vi "Recipe XML Editor.vi"(11 "TopLevel In":refnum<class "TopLevel.lvclass">) -> (3 "TopLevel out":refnum<class "TopLevel.lvclass">)   [LabVIEW 2022 SP3, in "TopLevel.lvclass"]
uses:
  TopLevel.lvclass
  Common/Controls/DLP2RecipeV2.ctl
panel:
  in  "Save Data to Recipe XML":bool
  in  "DLP":T1
  in  "Read Recipe XML":bool
  in  "Recipe XML File Path":path
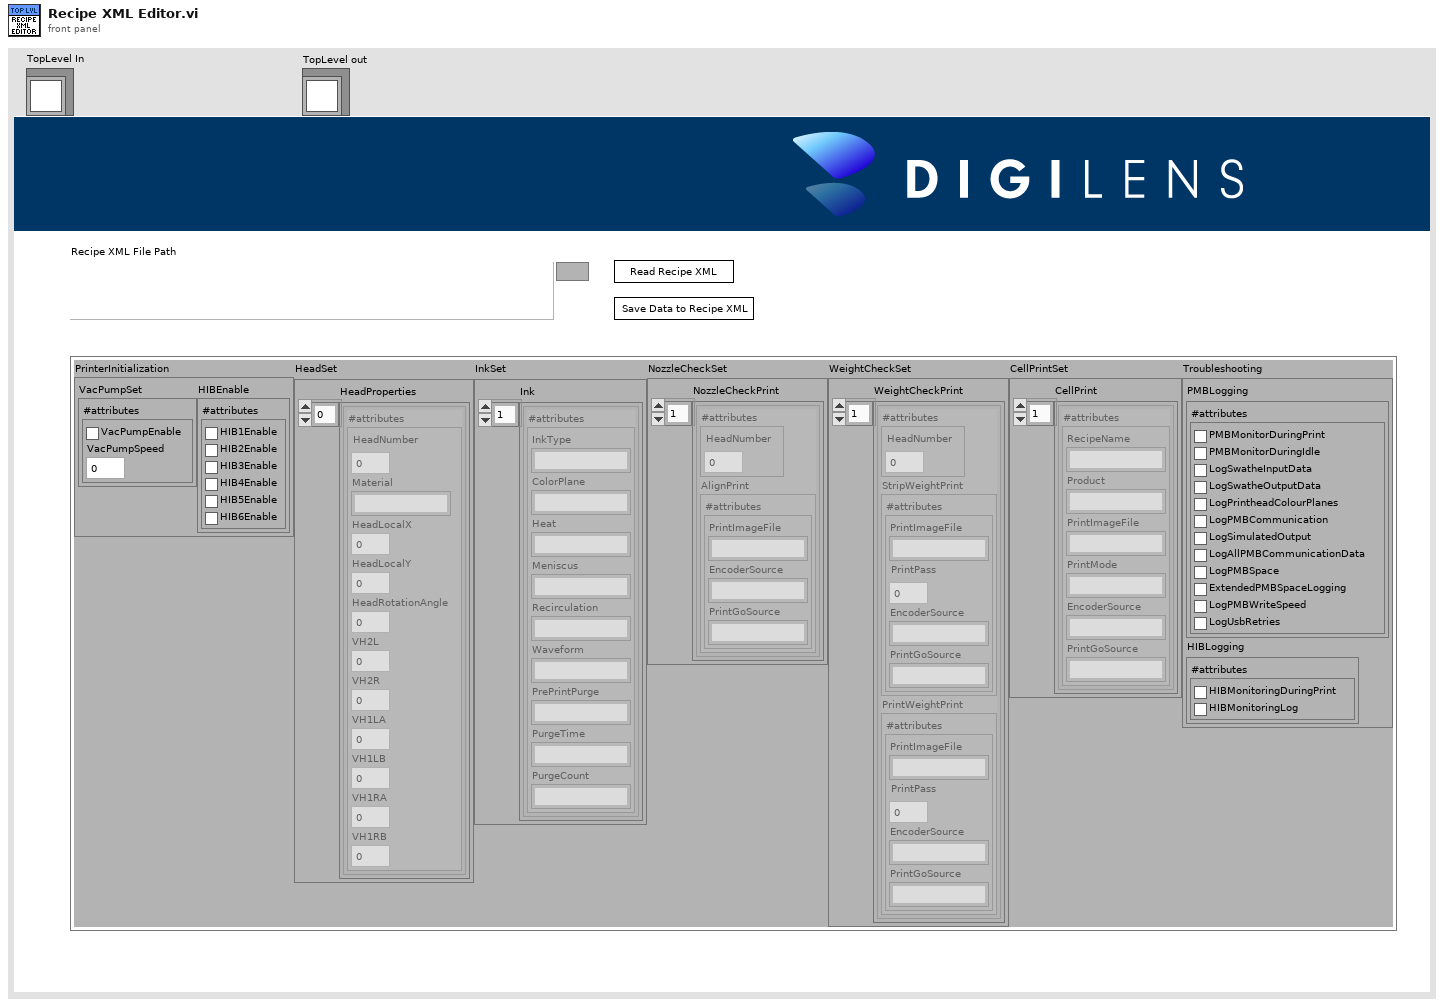
[diagram p1: front panel]
types:
  T1 = typedef "DLP2RecipeV2.ctl" = cluster{"PrinterInitialization":cluster{"VacPumpSet":cluster{"#attributes":cluster{"VacPumpEnable":bool, "VacPumpSpeed":dbl}}, "HIBEnable":cluster{"#attributes":cluster{"HIB1Enable":bool, "HIB2Enable":bool, "HIB3Enable":bool, "HIB4Enable":bool, "HIB5Enable":bool, "HIB6Enable":bool}}}, "HeadSet":cluster{"HeadProperties":cluster{"#attributes":cluster{"HeadNumber":u8, "Material":string, "HeadLocalX":dbl, "HeadLocalY":dbl, "HeadRotationAngle":dbl, "VH2L":dbl, "VH2R":dbl, "VH1LA":dbl, "VH1LB":dbl, "VH1RA":dbl, "VH1RB":dbl}}[]}, "InkSet":cluster{"Ink":cluster{"#attributes":cluster{"InkType":string, "ColorPlane":string, "Heat":string, "Meniscus":string, "Recirculation":string, "Waveform":string, "PrePrintPurge":string, "PurgeTime":string, "PurgeCount":string}}[]}, "NozzleCheckSet":cluster{"NozzleCheckPrint":cluster{"#attributes":cluster{"HeadNumber":u8}, "AlignPrint":cluster{"#attributes":cluster{"PrintImageFile":string, "EncoderSource":string, "PrintGoSource":string}}}[]}, "WeightCheckSet":cluster{"WeightCheckPrint":cluster{"#attributes":cluster{"HeadNumber":u8}, "StripWeightPrint":cluster{"#attributes":cluster{"PrintImageFile":string, "PrintPass":u8, "EncoderSource":string, "PrintGoSource":string}}, "PrintWeightPrint":cluster{"#attributes":cluster{"PrintImageFile":string, "PrintPass":u8, "EncoderSource":string, "PrintGoSource":string}}}[]}, "CellPrintSet":cluster{"CellPrint":cluster{"#attributes":cluster{"RecipeName":string, "Product":string, "PrintImageFile":string, "PrintMode":string, "EncoderSource":string, "PrintGoSource":string}}[]}, "Troubleshooting":cluster{"PMBLogging":cluster{"#attributes":cluster{"PMBMonitorDuringPrint":bool, "PMBMonitorDuringIdle":bool, "LogSwatheInputData":bool, "LogSwatheOutputData":bool, "LogPrintheadColourPlanes":bool, "LogPMBCommunication":bool, "LogSimulatedOutput":bool, "LogAllPMBCommunicationData":bool, "LogPMBSpace":bool, "ExtendedPMBSpaceLogging":bool, "LogPMBWriteSpeed":bool, "LogUsbRetries":bool}}, "HIBLogging":cluster{"#attributes":cluster{"HIBMonitoringDuringPrint":bool, "HIBMonitoringLog":bool}}}}
  T2 = enum32{"invalid app kind", "Development System", "Run Time System", "Student Edition", "Embedded LabVIEW", "Evaluation", "Custom"}
  T3 = enum32{"Invalid", "Standard", "Closed", "Hidden", "Minimized", "Maximized"}
  T4 = cluster{"Core":cluster{"Current VI Reference":refnum<vi>, "Close Panel on Exit?":bool}, "TopLevel In":refnum<class "TopLevel.lvclass">}
  T5 = cluster{"Current VI Reference":refnum<vi>, "Close Panel on Exit?":bool}
  T6 = typedef "TopLevel.lvclass/UserEvents.ctl" = cluster{"API Incoming Event":refnum<user-event>, "API Executed Event":refnum<user-event>, "API Return Event":refnum<user-event>, "Exit Event":refnum<user-event>, "StatusChanged":refnum<user-event>, "DLP GUI Config Changed":refnum<user-event>, "AppEvent":refnum<user-event>, "Login Event":refnum<user-event>, "HeadPrimeStatusEvent":refnum<user-event>}
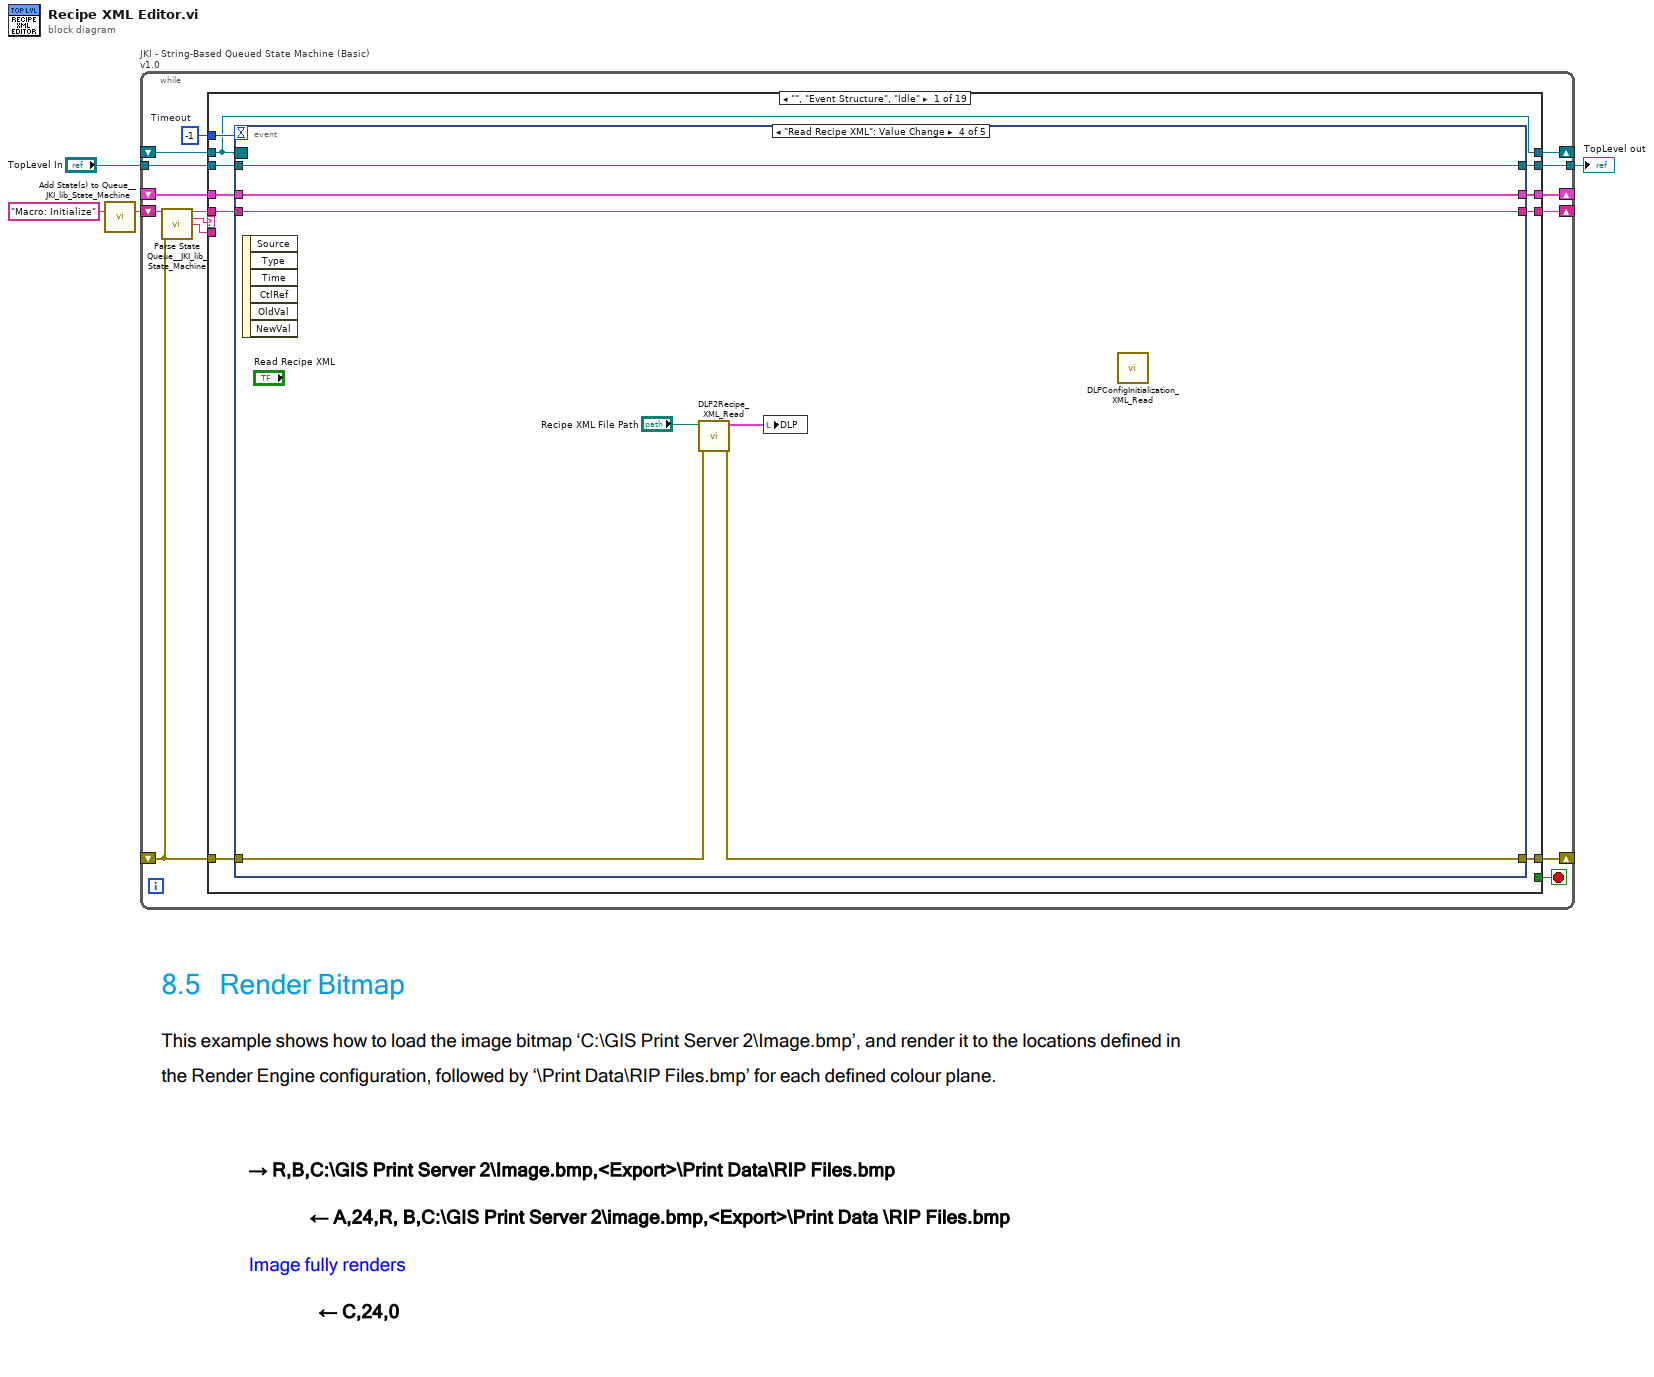
[diagram p0: block diagram]
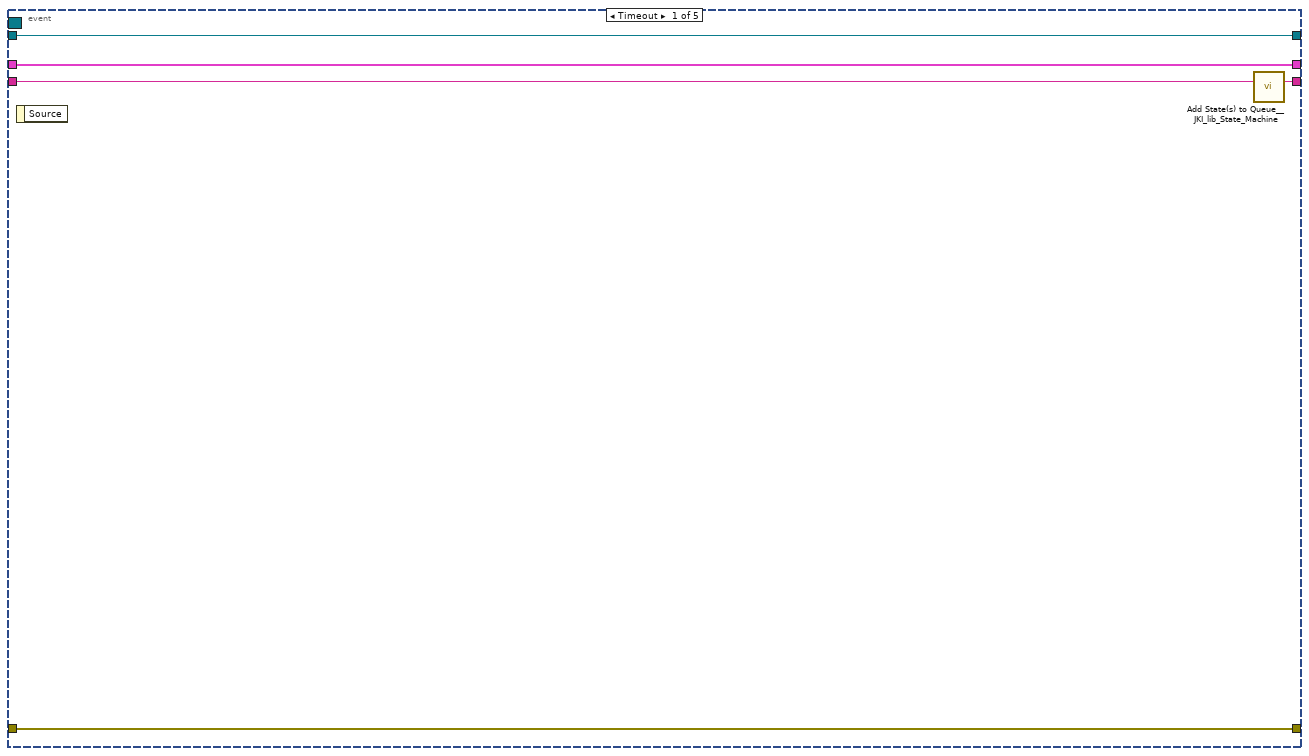
[diagram p2: hidden frame]
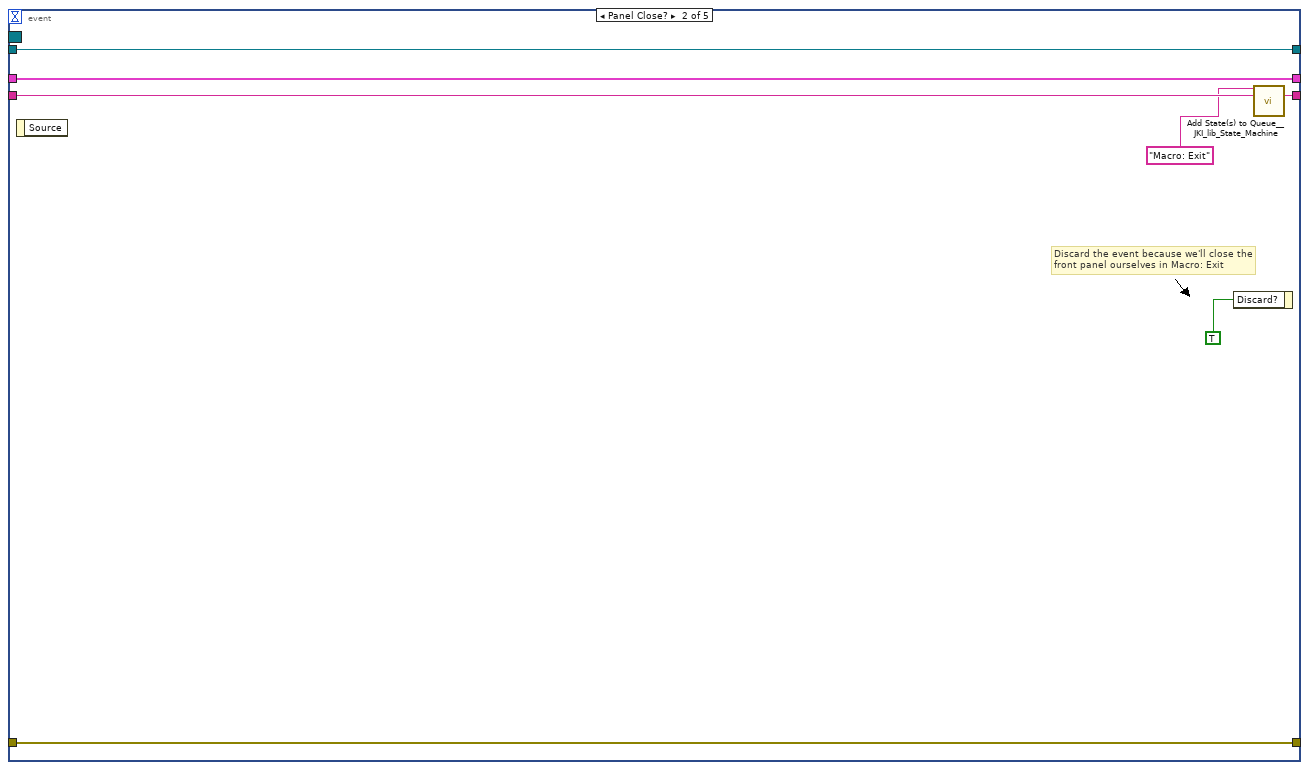
[diagram p3: hidden frame]
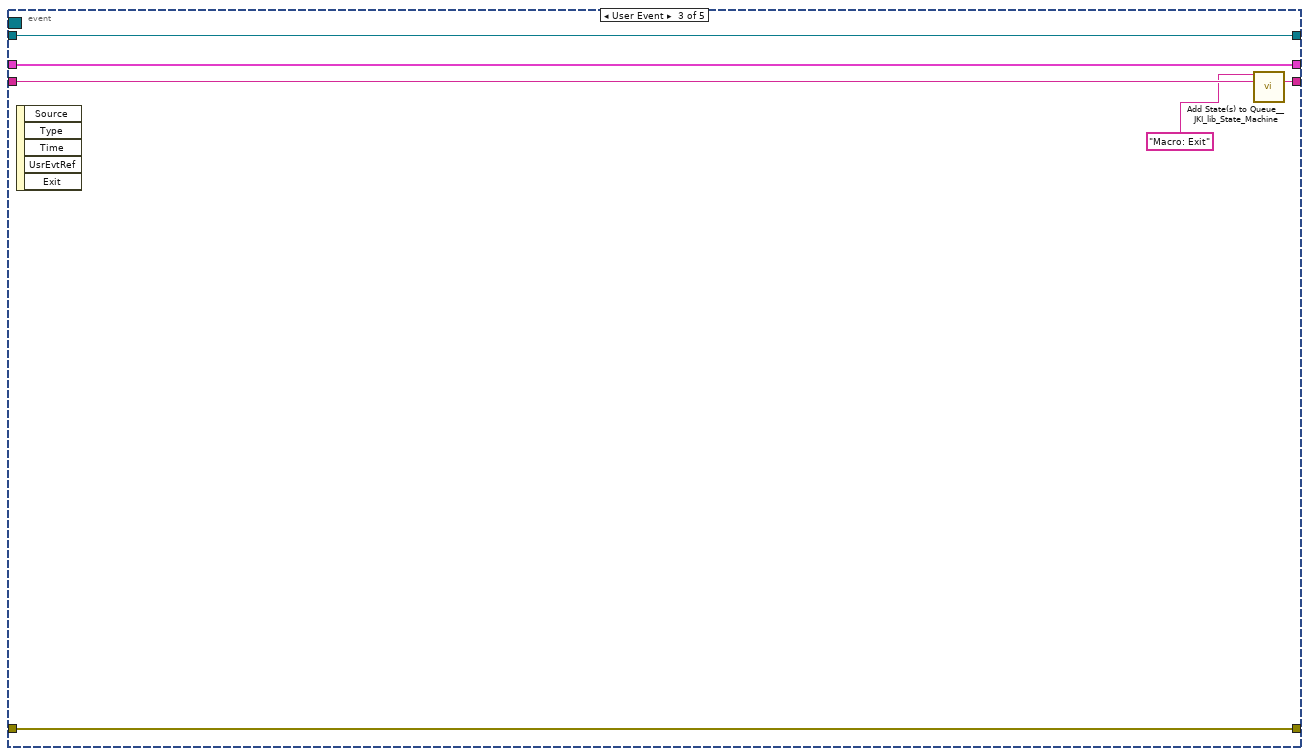
[diagram p4: hidden frame]
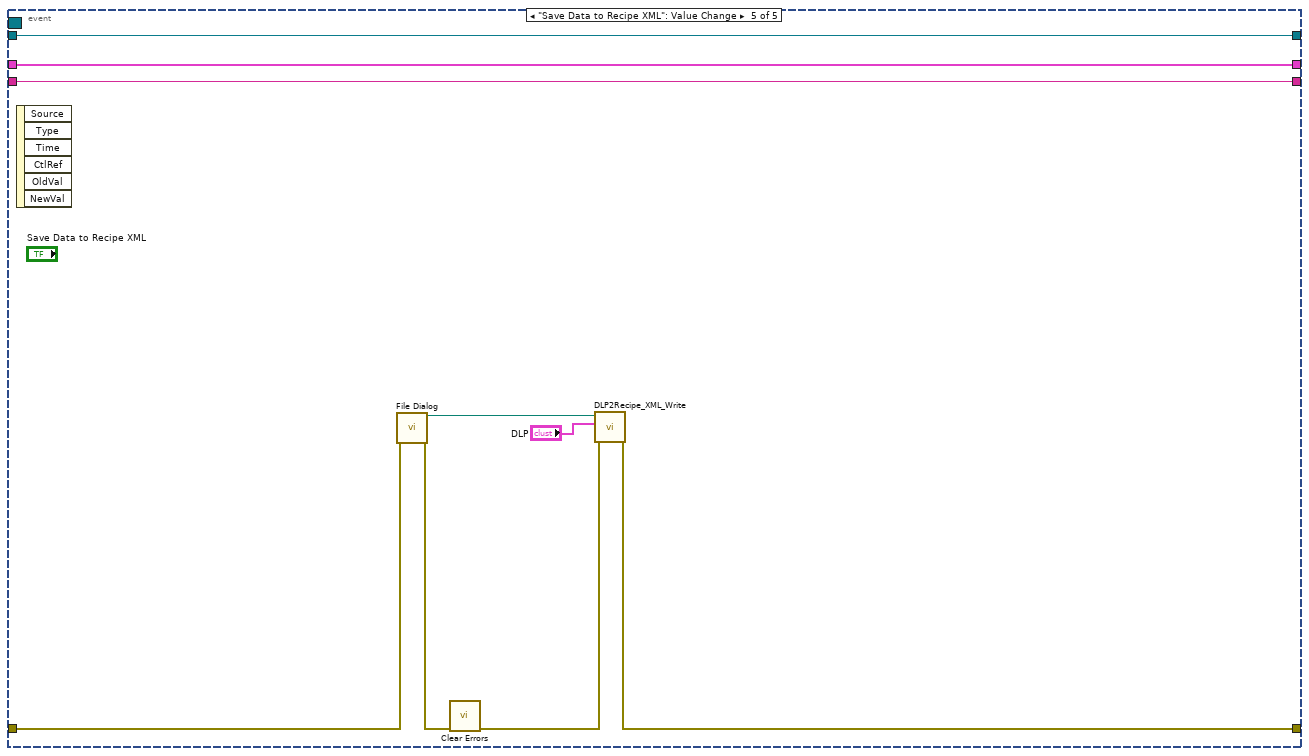
[diagram p5: hidden frame]
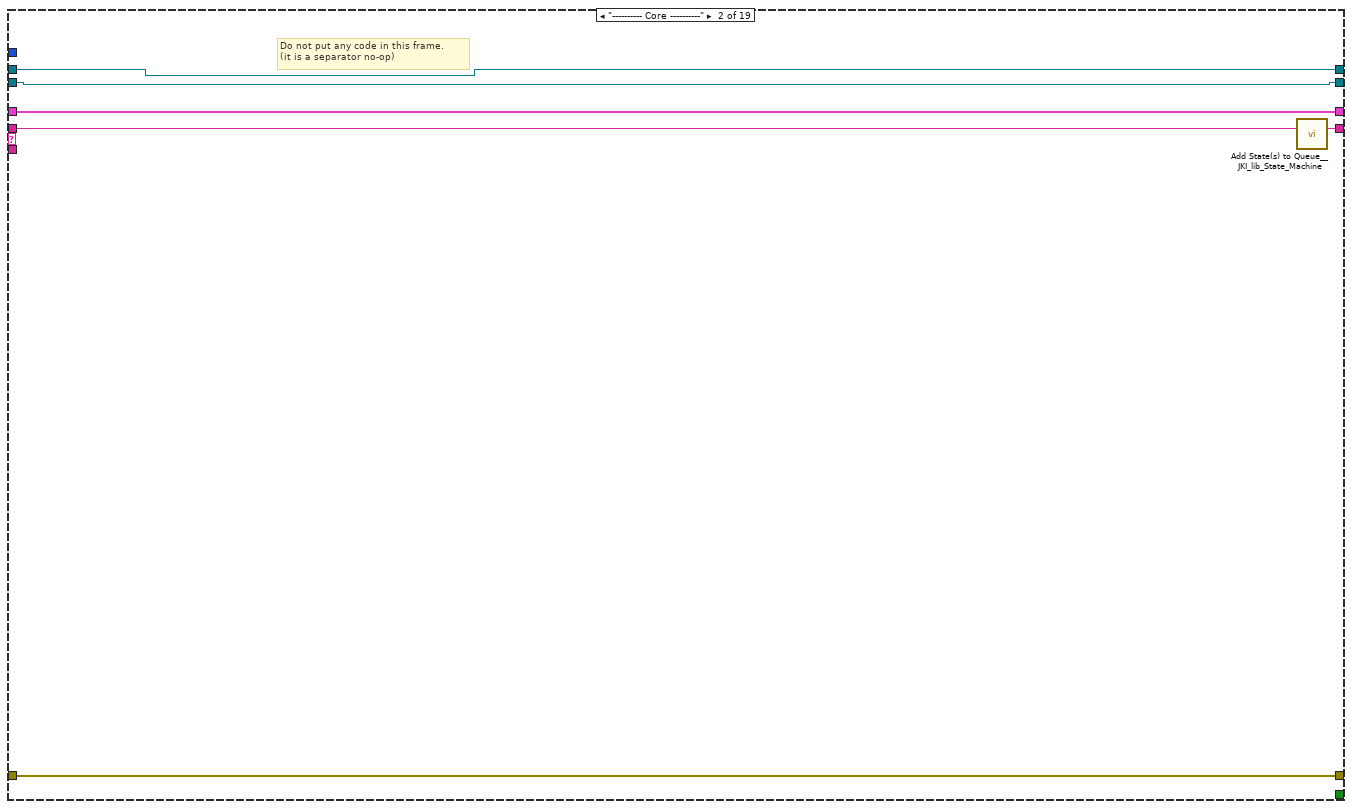
[diagram p6: hidden frame]
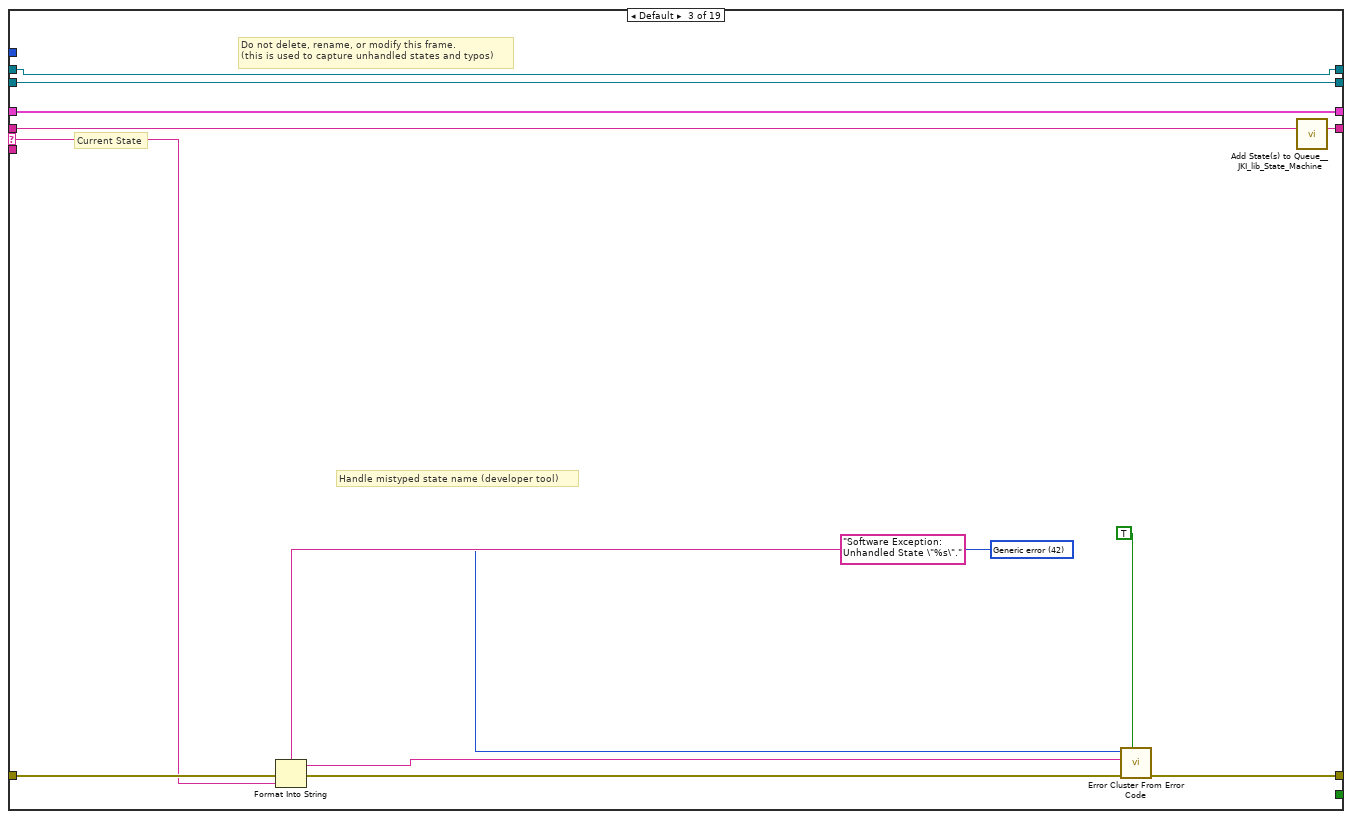
[diagram p7: hidden frame]
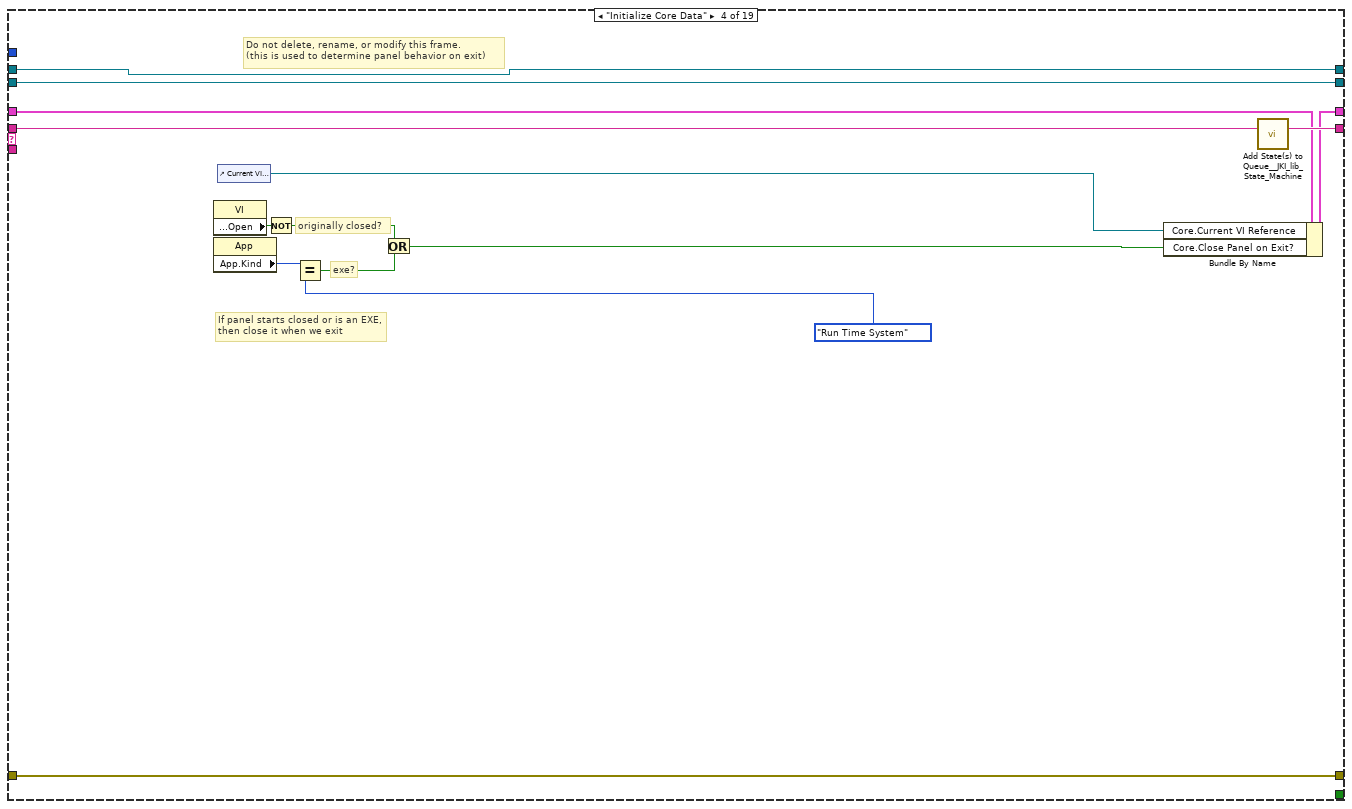
[diagram p8: hidden frame]
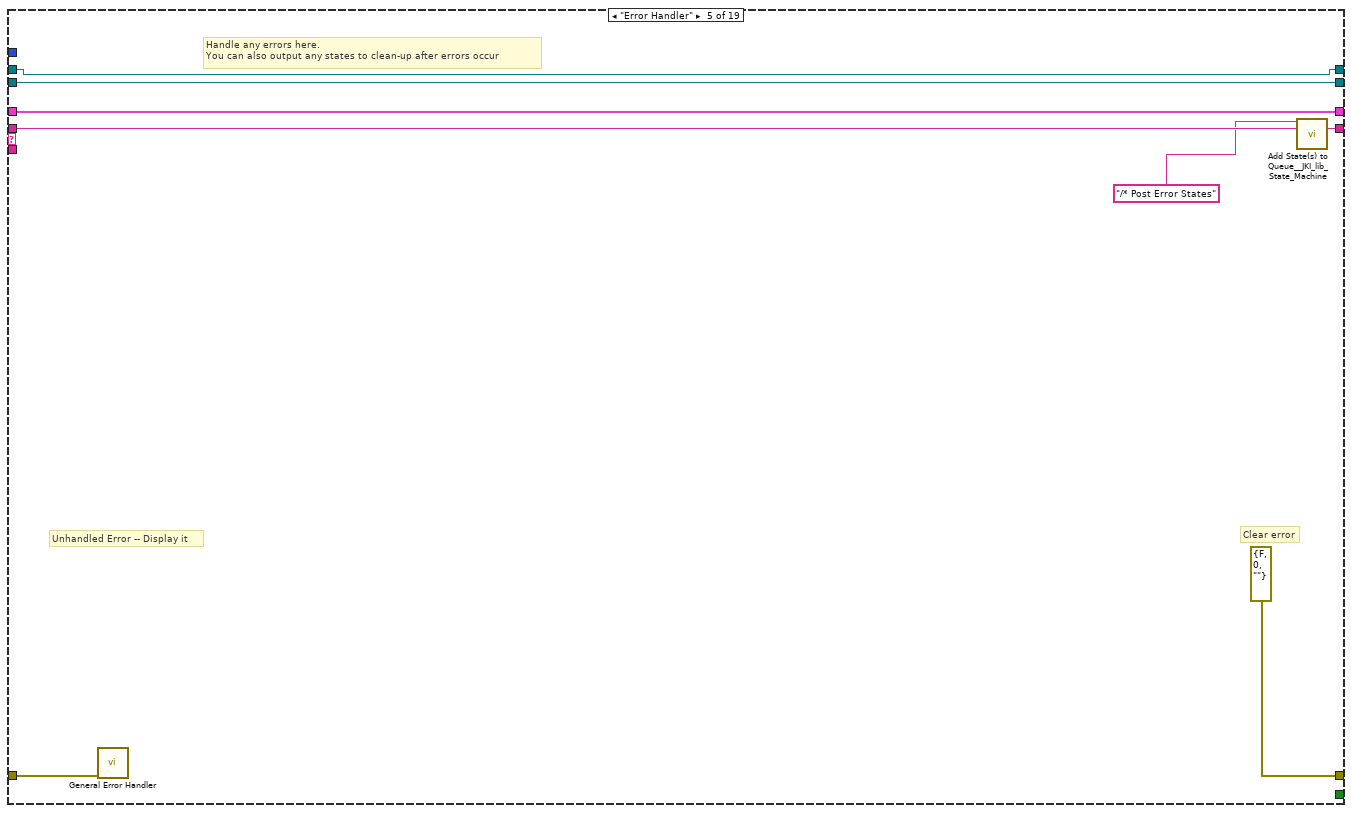
[diagram p9: hidden frame]
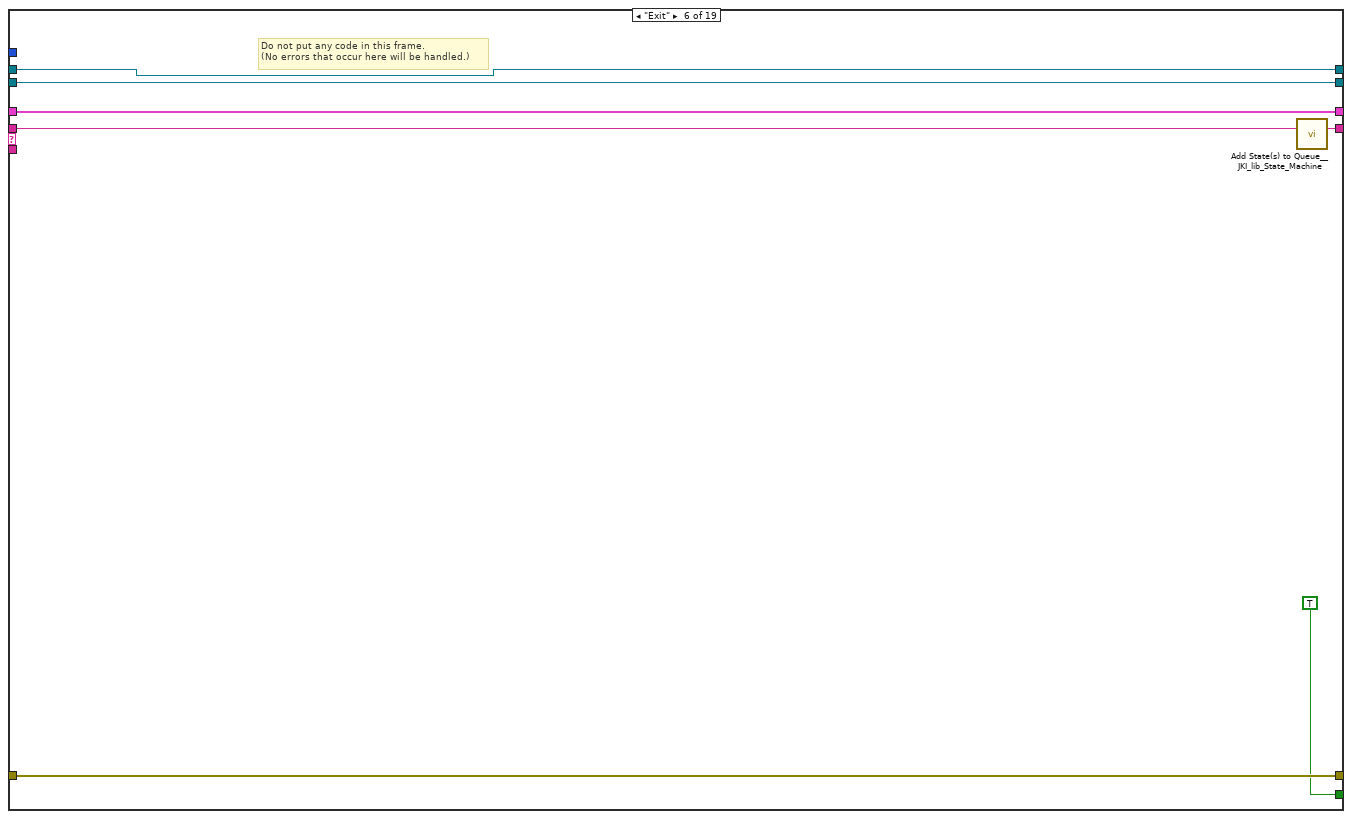
[diagram p10: hidden frame]
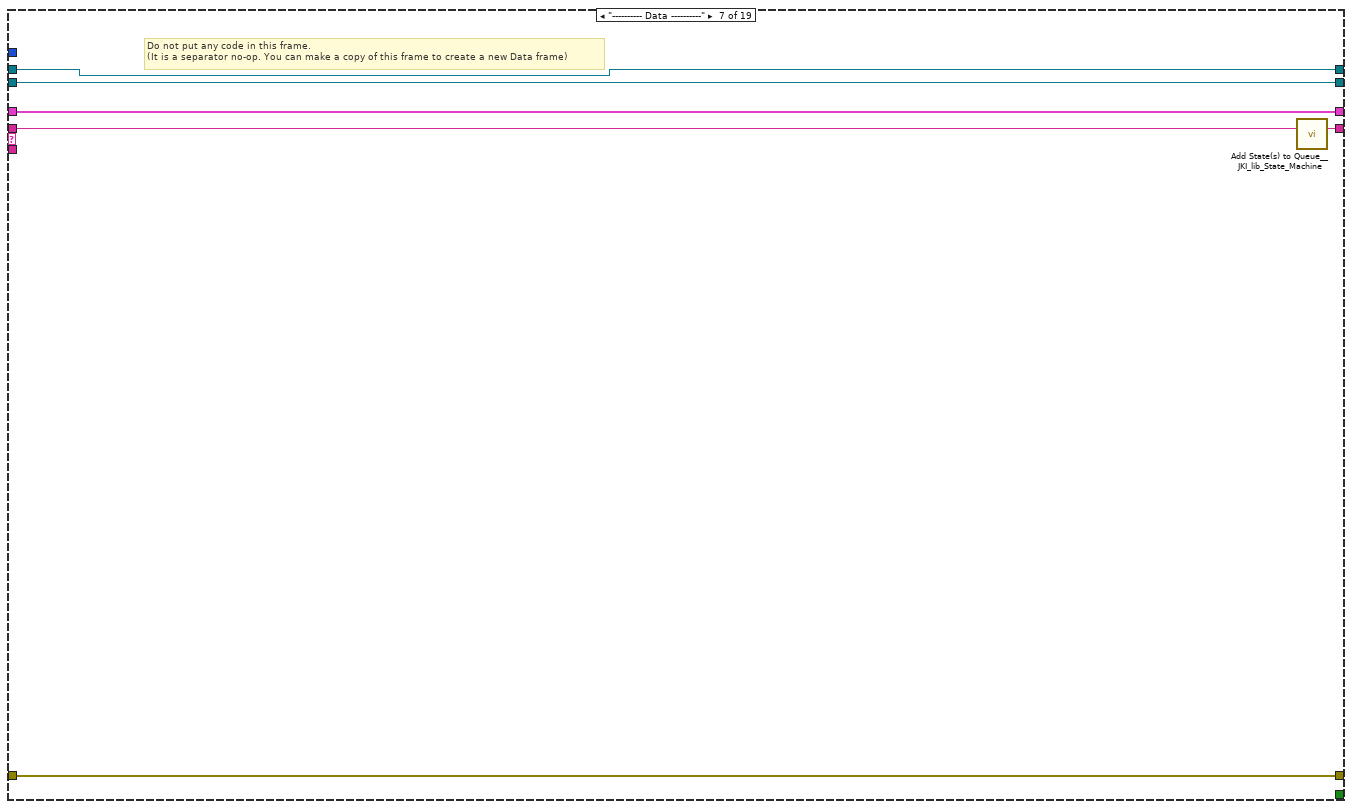
[diagram p11: hidden frame]
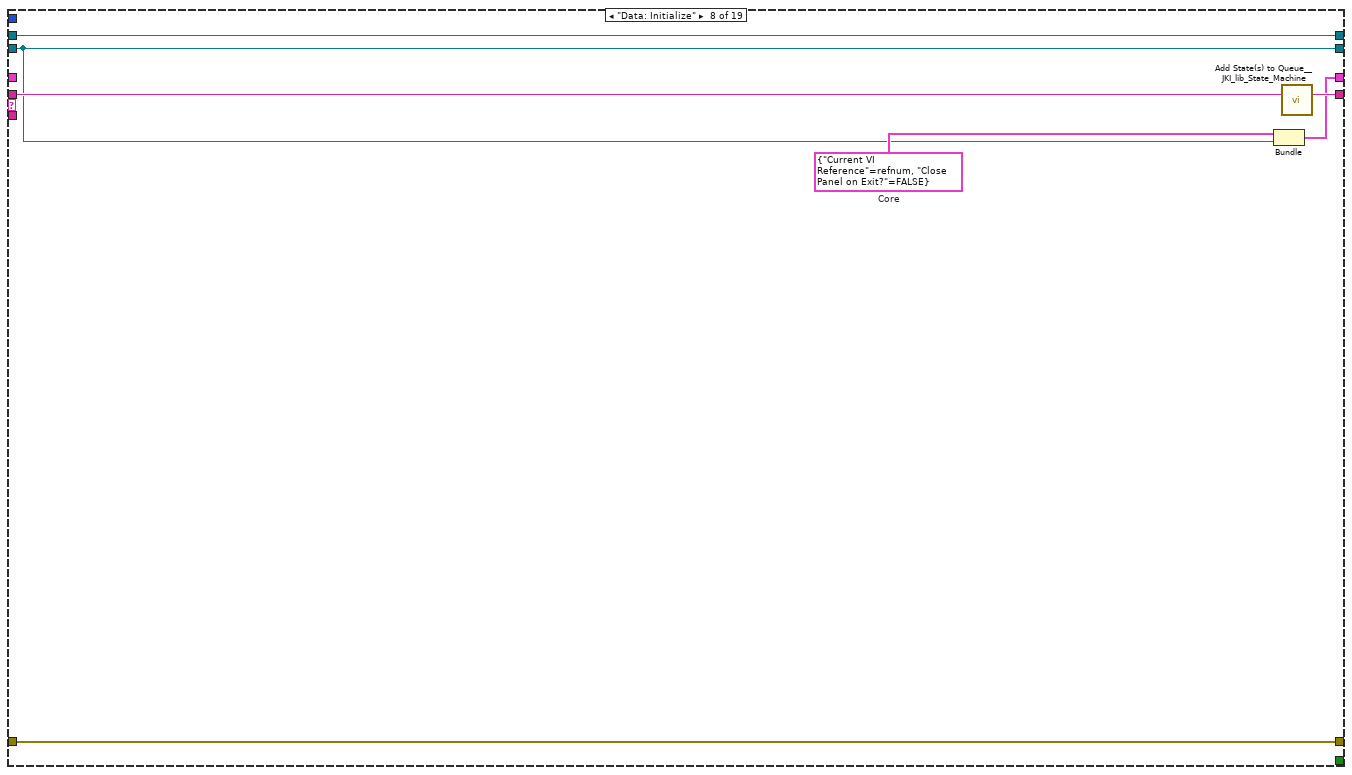
[diagram p12: hidden frame]
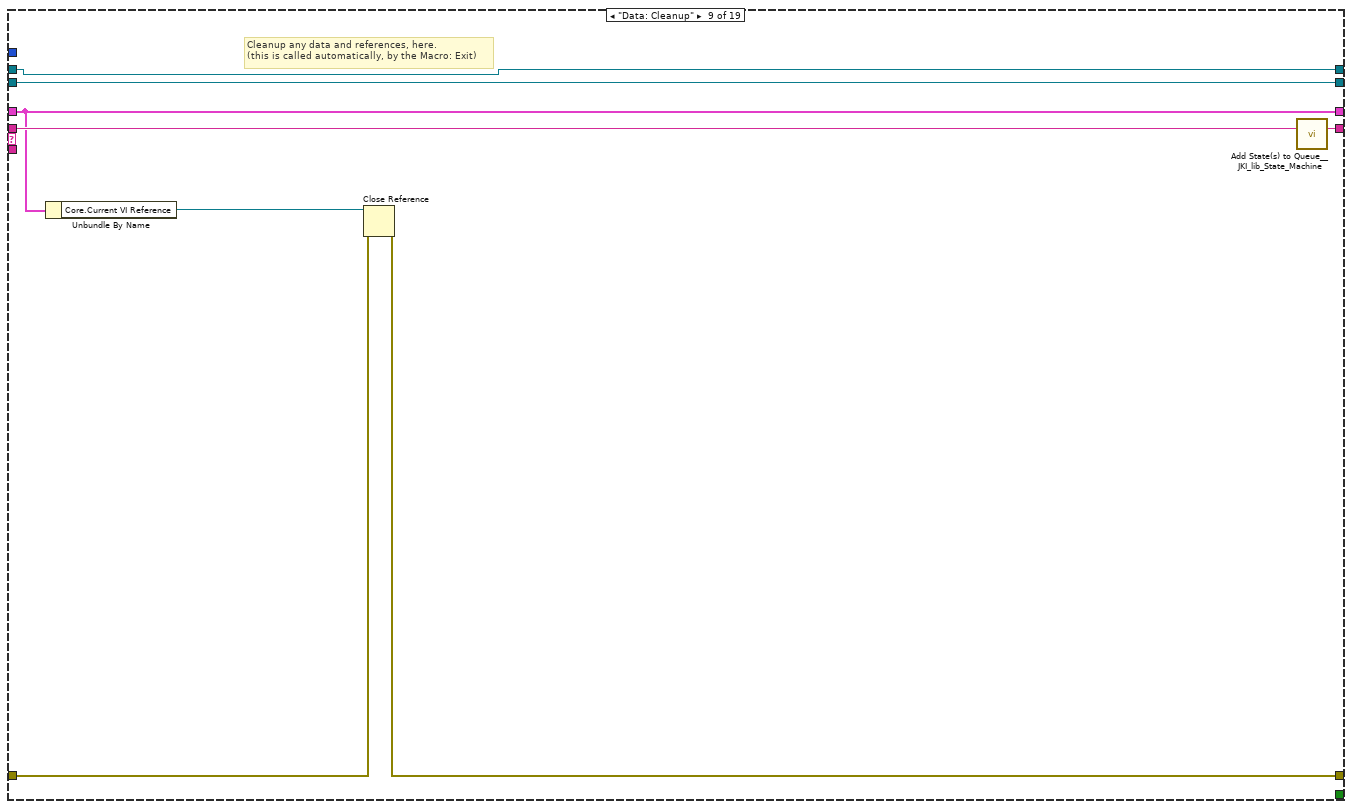
[diagram p13: hidden frame]
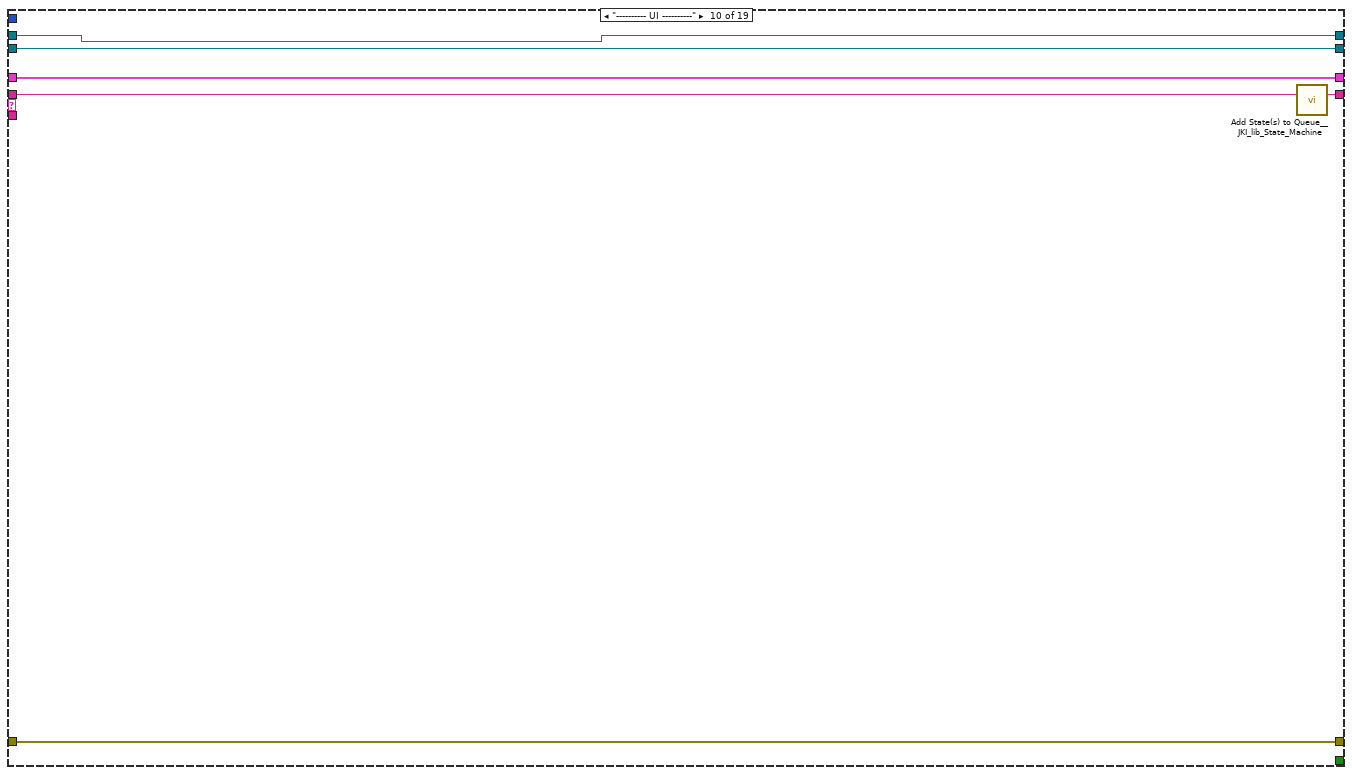
[diagram p14: hidden frame]
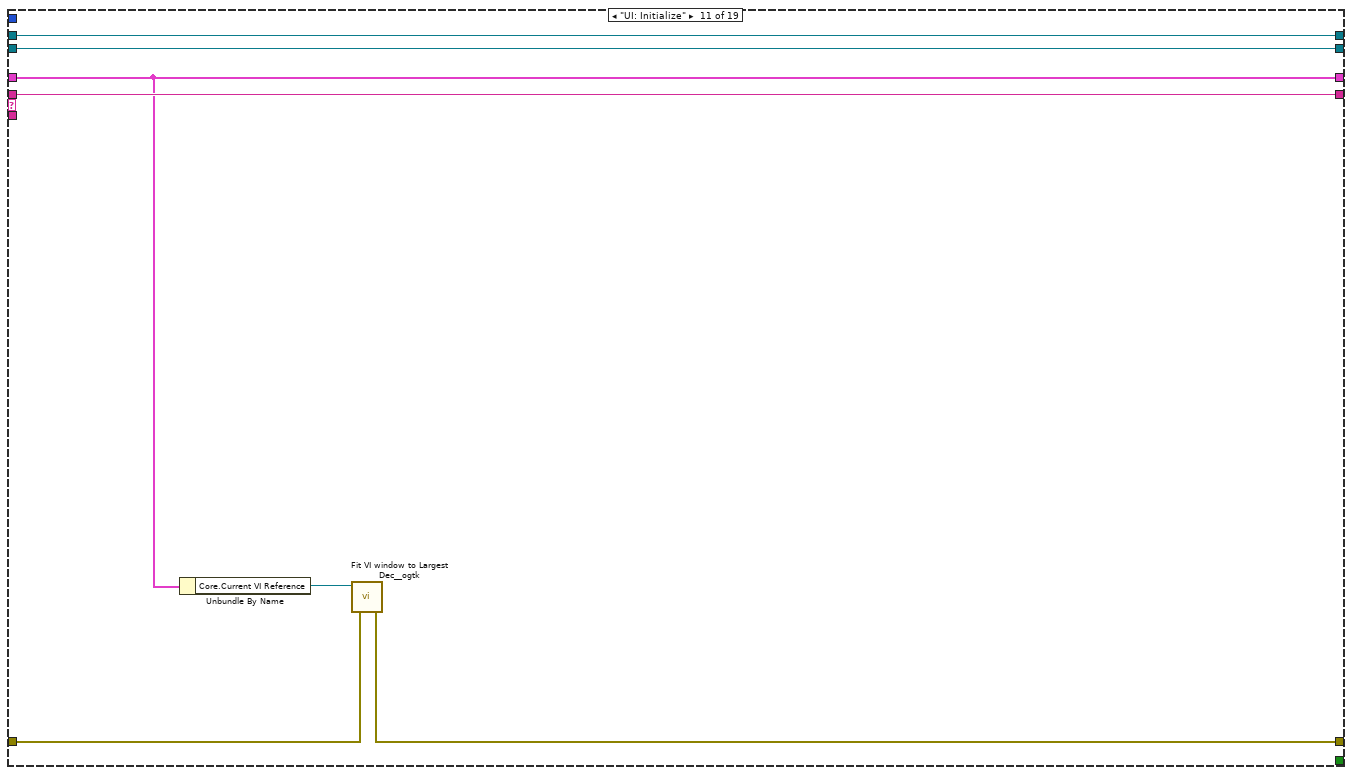
[diagram p15: hidden frame]
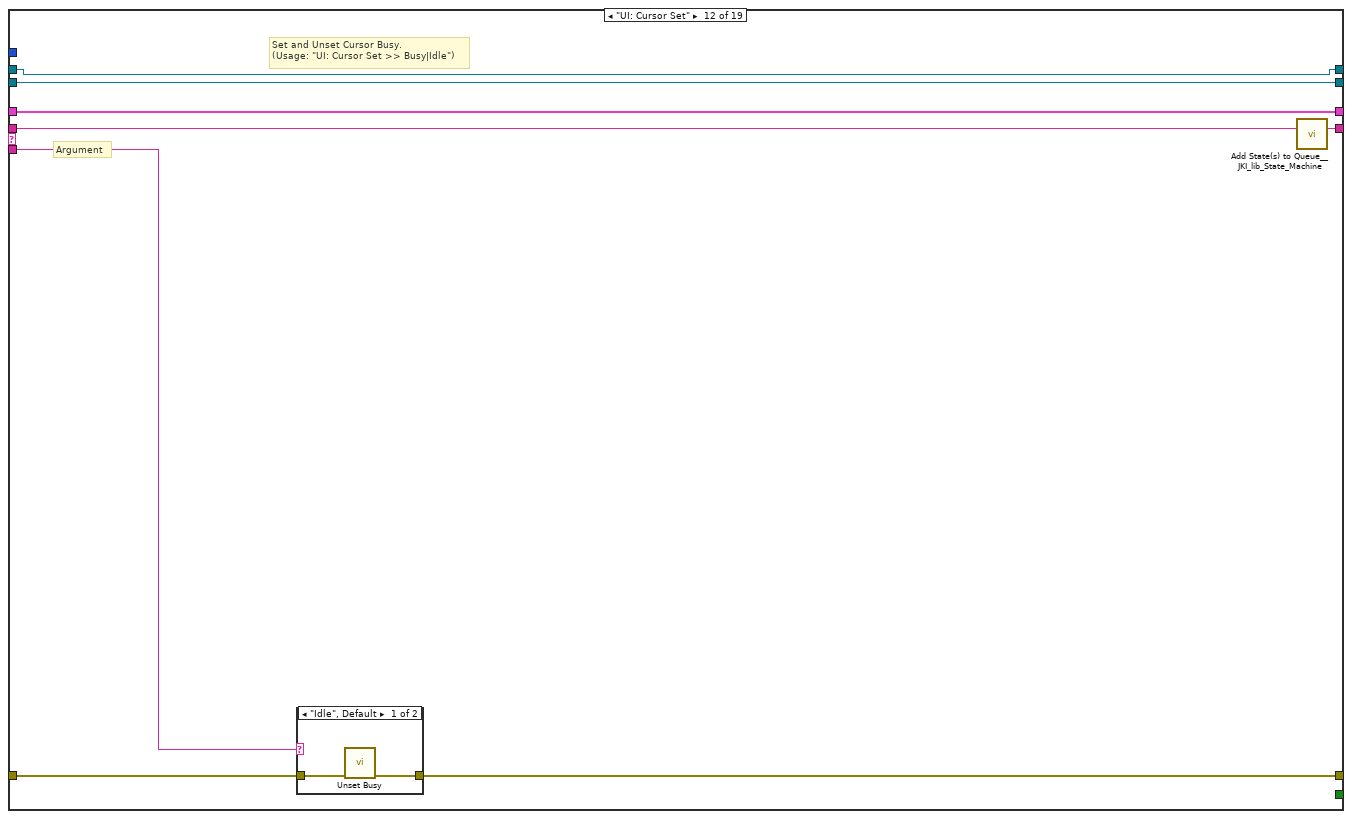
[diagram p16: hidden frame]
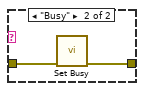
[diagram p17: hidden frame]
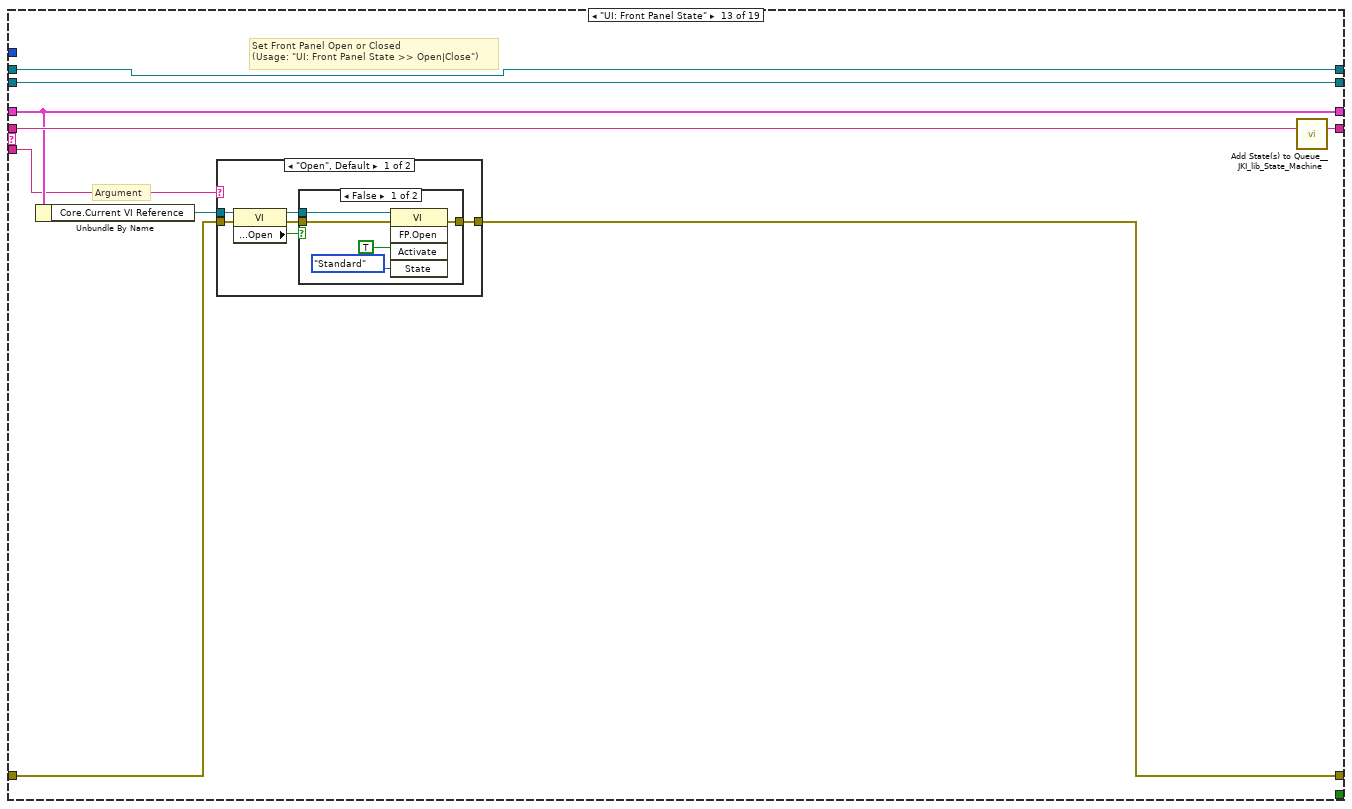
[diagram p18: hidden frame]
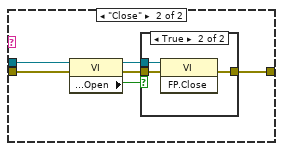
[diagram p20: hidden frame]
diagram:
  n1 = call <vilib>:"Add State(s) to Queue__JKI_lib_State_Machine.vi"("State(s) in (\"\")"="Macro: Initialize") -> ("States Out"=w4:string)  [unwired: 14 in]
  n2 = while "JKI - String-Based Queued State Machine (Basic) v1.0" {
    shift-right: [w12] -> _
    shift-left: _ -> [w11]
    shift-right: [w15] -> _
    shift-left: _ -> [w9]
    shift-right: [w14] -> _
    shift-left: w4 -> [w16]
    tunnel: "TopLevel In" -> [w8]
    tunnel: [w7] -> w1
    shift-right: [w6] -> _
    shift-left: _ -> [w5]
    stop <- w13 stop-if-true
    w10 = -1  # Timeout
    n3 = call <vilib>:"Parse State Queue__JKI_lib_State_Machine.vi"("State Queue"=w16, "Error In (no error)"=w9) -> ("Remaining States"=w18:string, "Current State"=w19:string, "Arguments"=w17:string)  [unwired: 11 in]
    n4 = case shown="\"\", \"Event Structure\", \"Idle\"" w19 {
      selector: w19 -> [_ _ w72 _ _ _ _ _ _ _ _ _ _ _ _ _ _ _ _]
      tunnel: w18 -> [w29 w69 w76 w96 w104 w111 w117 w124 w132 w138 w145 w153 w166 w194 w201 w213 w218 w227 w233]
      tunnel: w17 -> [_ _ _ _ _ _ _ _ _ _ _ w148 w160 _ _ _ _ _ _]
      tunnel: w11 -> [w27 w66 w74 w87 w101 w109 w114 _ w127 w135 w139 w151 w162 w191 w198 w203 w216 w225 w232]
      tunnel: [w26 w67 w78 w93 errorcluster {"status"=FALSE, "code"=0, "source"=""} ("error out") w108 w115 w119 w128 w136 w141 w149 w163 w192 w199 w202 w217 w222 w229] -> w15
      tunnel: w9 -> [w25 w67 w77 w93 w100 w108 w115 w119 w129 w136 w140 w150 w164 w192 w199 w202 w217 w219 w228]
      tunnel: [w28 w68 w75 w95 w103 w110 w116 w123 w131 w137 w145 w152 w165 w193 w200 w212 w218 w227 w233] -> w14
      tunnel: [_ _ _ _ _ TRUE _ _ _ _ _ _ _ _ _ _ _ _ _] -> w13
      tunnel: [w24 w66 w74 w94 w101 w109 w114 w122 w127 w135 w139 w151 w162 w191 w198 w203 w216 w225 w232] -> w12
      tunnel: w10 -> [w23 _ _ _ _ _ _ _ _ _ _ _ _ _ _ _ _ _ _]
      tunnel: w8 -> [w22 w65 w71 w84 w98 w106 w113 w118 w126 w134 w144 w147 w159 w190 w196 w204 w215 w226 w231]
      tunnel: [w21 w65 w71 w84 w98 w106 w113 w118 w126 w134 w144 w147 w159 w190 w196 w204 w215 w226 w231] -> w7
      tunnel: [w20 w64 w70 w83 w97 w105 w112 w120 w125 w133 w143 w146 w158 w189 w195 w205 w214 w224 w230] -> w6
      tunnel: w5 -> [w20 w64 w70 w83 w97 w105 w112 w120 w125 w133 w143 w146 w158 w189 w195 w205 w214 _ w230]
      frame "", "Event Structure", "Idle" {
        n5 = event shown="[3] \"Read Recipe XML\": Value Change" {
          selector: w20 -> [_ _ _ _ _]
          dyn-events: _ -> [_ _ _ _ _]
          timeout: w23 -> [_ _ _ _ _]
          tunnel: w29 -> [w34 w41 w47 w54 w63]
          tunnel: [w33 w40 w46 w54 w63] -> w28
          tunnel: w27 -> [w31 w36 w43 w53 w62]
          tunnel: [w32 w35 w42 w50 w59] -> w26
          tunnel: w25 -> [w32 w35 w42 w49 w55]
          tunnel: [w31 w36 w43 w53 w62] -> w24
          tunnel: w22 -> [w30 w37 w44 w52 w61]
          tunnel: [w30 w37 w44 w52 w61] -> w21
          event Timeout {
            n6 = event-data() -> ()  [unwired: 1 in, 1 out]
            n7 = call <vilib>:"Add State(s) to Queue__JKI_lib_State_Machine.vi"("State(s) in (\"\")"=w34) -> ("States Out"=w33:string)  [unwired: 14 in]
          }
          event Panel Close? {
            # "Discard the event because we'll close the front panel ourselves in Macro: Exit"
            n8 = event-data() -> ()  [unwired: 1 in, 1 out]
            n9 = event-data("Discard?"=TRUE) -> ()  [unwired: 1 in, 1 out]
            n10 = call <vilib>:"Add State(s) to Queue__JKI_lib_State_Machine.vi"("State(s) in Front (\"\")"="Macro: Exit", "State(s) in (\"\")"=w41) -> ("States Out"=w40:string)  [unwired: 13 in]
          }
          event User Event {
            n11 = event-data() -> ()  [unwired: 1 in, 5 out]
            n12 = call <vilib>:"Add State(s) to Queue__JKI_lib_State_Machine.vi"("State(s) in Front (\"\")"="Macro: Exit", "State(s) in (\"\")"=w47) -> ("States Out"=w46:string)  [unwired: 13 in]
          }
          event "Read Recipe XML": Value Change {
            n13 = event-data() -> ()  [unwired: 1 in, 6 out]
            n14 = call "DLP2Recipe_XML_Read.vi"("error in (no error)"=w49, "Recipe XML File Path"="Recipe XML File Path") -> ("error out"=w50:errorcluster, "data"=w48:T1)  [unwired: 8 in]
            n15 = local write "DLP"(w48) -> ()
            n16 = call "DLPConfigInitialization_XML_Read.vi"() -> ()  [unwired: 10 in, 2 out]
          }
          event "Save Data to Recipe XML": Value Change {
            n17 = event-data() -> ()  [unwired: 1 in, 6 out]
            n18 = call "File Dialog"("error in"=w55) -> ("selected path"=w58:path, "error out"=w57:errorcluster)  [unwired: 11 in, 2 out]
            n19 = call <vilib>:"Clear Errors.vi"("error in (no error)"=w57) -> ("error out"=w56:errorcluster)  [unwired: 5 in, 1 out]
            n20 = call "DLP2Recipe_XML_Write.vi"("error in (no error)"=w56, "data"="DLP", "Recipe XML File Path"=w58) -> ("error out"=w59:errorcluster)  [unwired: 7 in, 1 out]
          }
        }
      }
      frame "---------- Core ----------" {
        # "Do not put any code in this frame.\n(it is a separator no-op)"
        n21 = call <vilib>:"Add State(s) to Queue__JKI_lib_State_Machine.vi"("State(s) in (\"\")"=w69) -> ("States Out"=w68:string)  [unwired: 14 in]
      }
      frame Default {
        w81 = 42 items=["No error", "Argument error", "Memory is full", "Out of zone", "End of file", "File already open", "Generic file I/O error", "File not found", "File permission error", "Disk is full", "Duplicate path", "Too many files open", "System feature not enabled", "Resource file not found", "Cannot add resource", "Resource not found", "Image not found", "Image memory error", "Pen does not exist", "Config type invalid", "Config token not found", "Config parse error", "Config memory error", "Bad external code format", "Bad external code offset", "External code not present", "Null window", "Destroy window error", "Null menu", "Print aborted", "Bad print record", "Print driver error", "Windows error during printing", "Memory error during printing", "Print dialog error", "Generic print error", "Invalid device refnum", "Device not found", "Device parameter error", "Device unit error", "Cannot open device", "Device call aborted", "Generic error", "Cancelled by user", "Object ID too low", "Object ID too high", "Object not in heap", "Unknown heap", "Unknown object (invalid DefProc)", "Unknown object (DefProc not in table)", "Message out of range", "Invalid (null) method", "Unknown message", "Manager call not supported", "Bad address", "Network operation in progress", "Network operation timed out", "Connection is busy", "Network attribute not supported", "Network error", "Address in use", "System out of memory", "Connection aborted", "Connection refused", "Not connected", "Already connected", "Connection closed", "Initialization error (interapplication manager)", "Bad occurrence", "Wait on unbound occurrence handler", "Occurrence queue overflow", "Datalog type conflict", "Unused", "Unrecognized type (interapplication manager)", "Memory corrupt", "Failed to make temporary DLL", "Old CIN version", "Drag socket not found", "Failed to load drop-object", "Failed to register OLE object", "Failed to release OLE object", "Format specifier type mismatch", "Unknown format specifier", "Too few format specifiers", "Too many format specifiers", "Scan failed", "Newer CIN version", "Error converting to variant", "Runtime menu error", "Password tampered", "Variant attribute not found", "Incompatible variant data type", "Event data is not available", "Event Store is not present", "Occurrence is not found", "Event Queue is not created", "Event info is not available", "Refnum passed is NULL", "Error retrieving Class GUID", "Error retrieving CoClass GUID", "Error retrieving TypeLib GUID.", "Bad built application magic bytes.", "Specific driver is different from the specific driver associated with the Logical Name.", "There is no session opened to the class driver.", "Max Error", "MAX - Error with config objects", "MAX - Error loading configuration", "MAX - Group not supported"]
        # "Current State"
        # "Do not delete, rename, or modify this frame.\n(this is used to capture unhandled states and typos)"
        # "Handle mistyped state name (developer tool)"
        n22 = Format Into String(format string="Software Exception: Unhandled State \"%s\"." ("message"), error in=w77, w72) -> (resulting string=w80:string, error out=w79:errorcluster)  [unwired: 1 in]
        n23 = call <vilib>:"Error Cluster From Error Code.vi"("show call chain? (False)"=TRUE, "error in (no error)"=w79, "error message (\"\")"=w80, "error code (0)"=w81) -> ("error out"=w78:errorcluster)  [unwired: 5 in]
        n24 = call <vilib>:"Add State(s) to Queue__JKI_lib_State_Machine.vi"("State(s) in (\"\")"=w76) -> ("States Out"=w75:string)  [unwired: 14 in]
      }
      frame "Initialize Core Data" {
        # "Do not delete, rename, or modify this frame.\n(this is used to determine panel behavior on exit)"
        # "originally closed?"
        # "exe?"
        # "If panel starts closed or is an EXE, then close it when we exit"
        n25 = property class="VI"() -> ("Front Panel.Open"=w92:bool)  [unwired: 2 in, 2 out]
        n26 = property class="App"() -> ("App.Kind"=w91:T2)  [unwired: 2 in, 2 out]
        n27 = control-ref of="Current VI Reference"() -> (w85:refnum<vi>)
        n28 = Not(x=w92) -> (.not. x?=w89:bool)
        n29 = Equal?(x=w91, y=T2."Run Time System" ("Application:Kind")) -> (x = y?=w88:bool)
        n30 = Or(x=w89, y=w88) -> (x .or. y?=w86:bool)
        n31 = Bundle By Name(cluster=w87, "Core.Current VI Reference"=w85, "Core.Close Panel on Exit?"=w86) -> (w94:T4)
        n32 = call <vilib>:"Add State(s) to Queue__JKI_lib_State_Machine.vi"("State(s) in (\"\")"=w96) -> ("States Out"=w95:string)  [unwired: 14 in]
      }
      frame "Error Handler" {
        # "Unhandled Error -- Display it"
        # "Handle any errors here.\nYou can also output any states to clean-up after errors occur"
        # "Clear error"
        n33 = call <vilib>:"General Error Handler.vi"("error in (no error)"=w100) -> ()  [unwired: 10 in, 5 out]
        n34 = call <vilib>:"Add State(s) to Queue__JKI_lib_State_Machine.vi"("State(s) in Front (\"\")"="/* Post Error States", "State(s) in (\"\")"=w104) -> ("States Out"=w103:string)  [unwired: 13 in]
      }
      frame "Exit" {
        # "Do not put any code in this frame.\n(No errors that occur here will be handled.)"
        n35 = call <vilib>:"Add State(s) to Queue__JKI_lib_State_Machine.vi"("State(s) in (\"\")"=w111) -> ("States Out"=w110:string)  [unwired: 14 in]
      }
      frame "---------- Data ----------" {
        # "Do not put any code in this frame.\n(It is a separator no-op. You can make a copy of this frame to create a new Data frame)"
        n36 = call <vilib>:"Add State(s) to Queue__JKI_lib_State_Machine.vi"("State(s) in (\"\")"=w117) -> ("States Out"=w116:string)  [unwired: 14 in]
      }
      frame "Data: Initialize" {
        w121 = T5 {"Current VI Reference"=refnum, "Close Panel on Exit?"=FALSE}  # Core
        n37 = Bundle("Core"=w121, "TopLevel In"=w118) -> (w122:T4)  [unwired: 1 in]
        n38 = call <vilib>:"Add State(s) to Queue__JKI_lib_State_Machine.vi"("State(s) in (\"\")"=w124) -> ("States Out"=w123:string)  [unwired: 14 in]
      }
      frame "Data: Cleanup" {
        # "Cleanup any data and references, here.\n(this is called automatically, by the Macro: Exit)"
        n39 = Unbundle By Name(w127) -> ("Core.Current VI Reference"=w130:refnum<vi>)
        n40 = Close Reference(reference=w130, error in (no error)=w129) -> (error out=w128:errorcluster)
        n41 = call <vilib>:"Add State(s) to Queue__JKI_lib_State_Machine.vi"("State(s) in (\"\")"=w132) -> ("States Out"=w131:string)  [unwired: 14 in]
      }
      frame "---------- UI ----------" {
        n42 = call <vilib>:"Add State(s) to Queue__JKI_lib_State_Machine.vi"("State(s) in (\"\")"=w138) -> ("States Out"=w137:string)  [unwired: 14 in]
      }
      frame "UI: Initialize" {
        n43 = Unbundle By Name(w139) -> ("Core.Current VI Reference"=w142:refnum<vi>)
        n44 = call <userlib>:"Fit VI window to Largest Dec__ogtk.vi"("error in (no error)"=w140, "VI Ref (calling VI)"=w142) -> ("error out"=w141:errorcluster)  [unwired: 4 in, 1 out]
      }
      frame "UI: Cursor Set" {
        # "Argument"
        # "Set and Unset Cursor Busy.\n(Usage: \"UI: Cursor Set >> Busy|Idle\")"
        n45 = case shown="\"Idle\", Default" w148 {
          tunnel: w150 -> [w155 w157]
          tunnel: [w154 w156] -> w149
          frame "Idle", Default {
            n46 = call <vilib>:"Unset Busy.vi"("error in (no error)"=w155) -> ("error out"=w154:errorcluster)  [unwired: 10 in]
          }
          frame "Busy" {
            n47 = call <vilib>:"Set Busy.vi"("error in (no error)"=w157) -> ("error out"=w156:errorcluster)  [unwired: 9 in, 1 out]
          }
        }
        n48 = call <vilib>:"Add State(s) to Queue__JKI_lib_State_Machine.vi"("State(s) in (\"\")"=w153) -> ("States Out"=w152:string)  [unwired: 14 in]
      }
      frame "UI: Front Panel State" {
        # "Argument"
        # "Set Front Panel Open or Closed\n(Usage: \"UI: Front Panel State >> Open|Close\")"
        n49 = Unbundle By Name(w162) -> ("Core.Current VI Reference"=w161:refnum<vi>)
        n50 = case shown="\"Open\", Default" w160 {
          tunnel: w164 -> [w170 w183]
          tunnel: [w172 w184] -> w163
          tunnel: w161 -> [w171 w181]
          frame "Open", Default {
            n51 = property class="VI"(reference=w171, error in=w170) -> (reference out=w168:refnum<vi>, error out=w169:errorcluster, "Front Panel.Open"=w167:bool)
            n52 = case shown="False" w167 {
              tunnel: [w175 w178] -> w172
              tunnel: w169 -> [w174 w178]
              tunnel: w168 -> [w173 _]
              frame False {
                n53 = invoke class="VI" method="FP.Open"(reference=w173, error in=w174, "Activate"=TRUE, "State"=T3."Standard") -> (error out=w175:errorcluster)  [unwired: 1 in, 4 out]
              }
              frame True {
              }
            }
          }
          frame "Close" {
            n54 = property class="VI"(reference=w181, error in=w183) -> (reference out=w180:refnum<vi>, error out=w182:errorcluster, "Front Panel.Open"=w179:bool)
            n55 = case shown="True" w179 {
              tunnel: [w185 w188] -> w184
              tunnel: w182 -> [w185 w187]
              tunnel: w180 -> [_ w186]
              frame False {
              }
              frame True {
                n56 = invoke class="VI" method="FP.Close"(reference=w186, error in=w187) -> (error out=w188:errorcluster)  [unwired: 1 in, 2 out]
              }
            }
          }
        }
        n57 = call <vilib>:"Add State(s) to Queue__JKI_lib_State_Machine.vi"("State(s) in (\"\")"=w166) -> ("States Out"=w165:string)  [unwired: 14 in]
      }
      frame "---------- Macro ----------" {
        # "Do not put any code in this frame.\n(It is a separator no-op. You can make a copy of this frame to create a new Macro frame)"
        n58 = call <vilib>:"Add State(s) to Queue__JKI_lib_State_Machine.vi"("State(s) in (\"\")"=w194) -> ("States Out"=w193:string)  [unwired: 14 in]
      }
      frame "Macro: Initialize" {
        n59 = call <vilib>:"Add State(s) to Queue__JKI_lib_State_Machine.vi"("State(s) in Front (\"\")"="Data: Initialize\nInitialize Core Data\nUI: Initialize\nEvents: Register Events\nUI: Front Panel State >> Open", "State(s) in (\"\")"=w201) -> ("States Out"=w200:string)  [unwired: 13 in]
      }
      frame "Macro: Exit" {
        # "Exit Macro\n(This is called once, when the VI exits)"
        n60 = Unbundle By Name(w203) -> ("Core.Close Panel on Exit?"=w211:bool)
        n61 = Select(t="UI: Front Panel State >> Close", s=w211, f="") -> (s? t:f=w208:string)
        n62 = call <vilib>:"Add State(s) to Queue__JKI_lib_State_Machine.vi"("State(s) in (\"\")"=w208, "State(s) at Back (\"\")"="Data: Cleanup\nEvents: Unregister Events\nExit") -> ("States Out"=w206:string)  [unwired: 13 in]
        n63 = call <vilib>:"Add State(s) to Queue__JKI_lib_State_Machine.vi"("State(s) in Front (\"\")"=w206, "State(s) in (\"\")"=w213) -> ("States Out"=w212:string)  [unwired: 13 in]
      }
      frame "----------Events ----------" {
        # "Template Separator\n(You can make a copy of, or modify, this frame)"
      }
      frame "Events: Register Events" {
        n64 = Unbundle By Name(w225) -> ("TopLevel In"=w223:refnum<class "TopLevel.lvclass">)
        n65 = call-dynamic "GetEvents_TopLevel.vi"("error in (no error)"=w219, "TopLevel in"=w223) -> ("error out"=w222:errorcluster, "UserEvents"=w221:T6)  [unwired: 7 in, 1 out]
        n66 = Unbundle By Name(w221) -> ("Exit Event"=w220:refnum<user-event>)
        n67 = register-events(w220) -> (reference out=w224:refnum<event-registration>)  [unwired: 2 in, 1 out]
      }
      frame "Events: Unregister Events" {
        n68 = Unregister For Events(event registration refnum=w230, error in=w228) -> (error out=w229:errorcluster)
      }
    }
  }
  "TopLevel out" <- w1
